vi "Wait For Motion Done.vi"(8 "error in (no error)":errorcluster, 9 "Mono2 Motor Pos":refnum<vi>, 10 "Axis":i32=1, 11 "VISA resource name":refnum<visa-resource-name>) -> (0 "error out":errorcluster, 3 "VISA resource name out":refnum<visa-resource-name>)   [LabVIEW 2019]
panel:
  in  "Mono2 Motor Pos":dbl caption="Motor Pos"
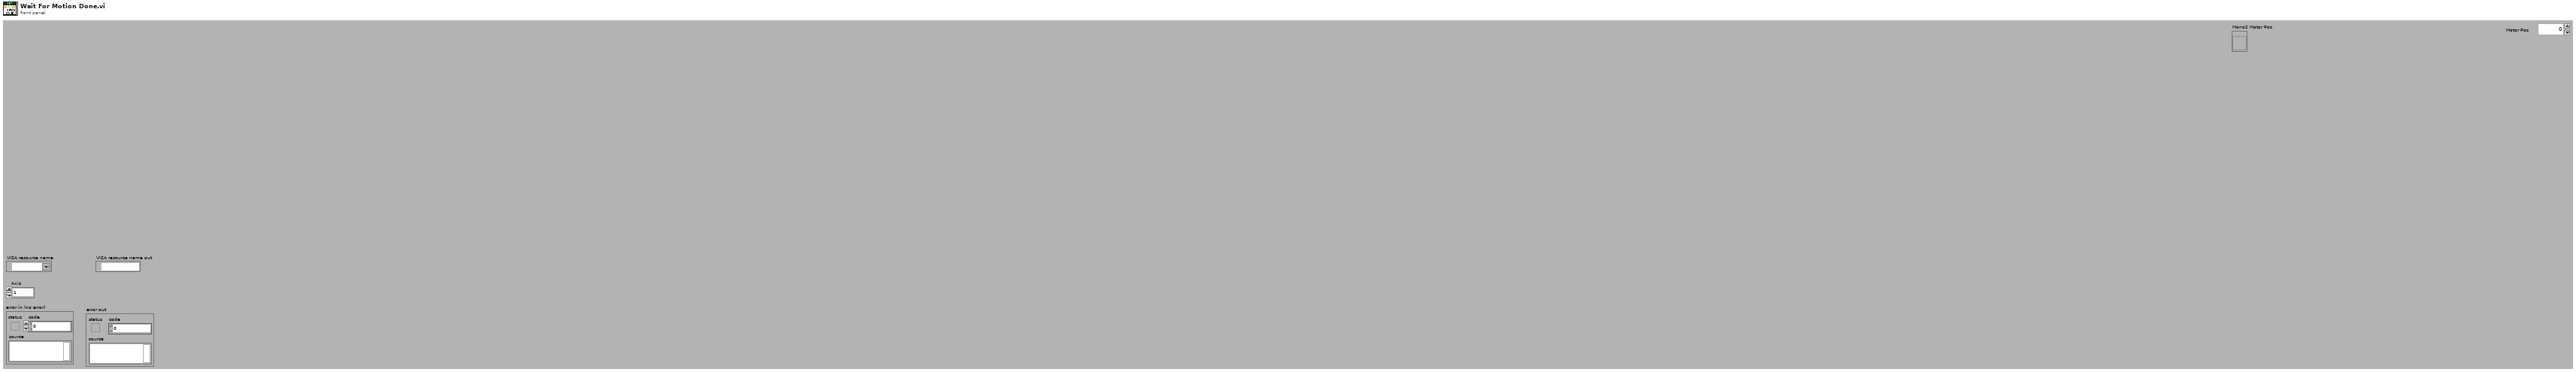
[diagram p1: front panel]
types:
  T1 = enum8{"Enabled", "Disabled", "Disabled and Grayed Out"}
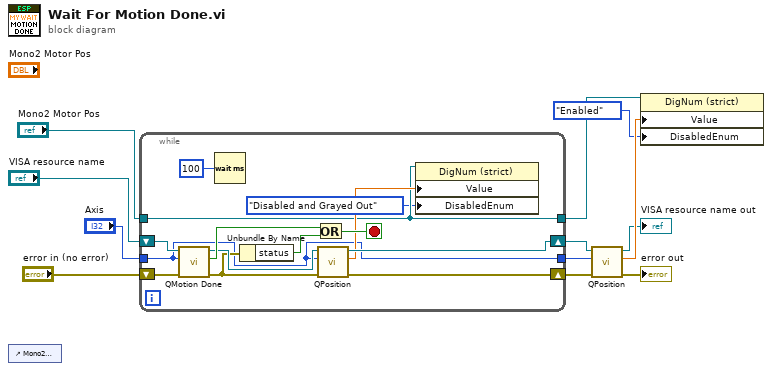
[diagram p0: block diagram]
diagram:
  n1 = control-ref of="Mono2 Motor Pos"() -> ()  [unwired: 1 out]
  n2 = while {
    shift-right: [w19] -> w4
    shift-left: "VISA resource name" -> [w26]
    shift-right: [w17] -> w7
    shift-left: "error in (no error)" -> [w25]
    tunnel: "Axis" -> [w15]
    tunnel: [w15] -> w8
    tunnel: [w14] -> w3
    tunnel: "Mono2 Motor Pos" -> [w14]
    stop <- w22 stop-if-true
    n3 = call "QMotion Done.vi"("error in (no error)"=w25, "Axis"=w15, "VISA resource name in"=w26) -> ("error out"=w18:errorcluster, "Motion Done?"=w23:bool, "VISA resource name out"=w20:refnum<visa-resource-name>)  [unwired: 6 in]
    n4 = Wait (ms)(milliseconds to wait=u32 100) -> ()  [unwired: 1 out]
    n5 = Unbundle By Name(w18) -> ("status"=w24:bool)
    n6 = Or(x=w23, y=w24) -> (x .or. y?=w22:bool)
    n7 = call "QPosition.vi"("error in (no error)"=w18, "Axis"=w15, "VISA resource name in"=w20) -> ("error out"=w17:errorcluster, "Position"=w16:dbl, "VISA resource name out"=w19:refnum<visa-resource-name>)  [unwired: 6 in]
    n8 = property class="DigNum (strict)"(reference=w14, "Value"=w16, "DisabledEnum"=T1."Disabled and Grayed Out" ("Disabled")) -> ()  [unwired: 1 in, 2 out]
  }
  n9 = call "QPosition.vi"("error in (no error)"=w7, "Axis"=w8, "VISA resource name in"=w4) -> ("error out"=→"error out":errorcluster, "Position"=w9:dbl, "VISA resource name out"=→"VISA resource name out":refnum<visa-resource-name>)  [unwired: 6 in]
  n10 = property class="DigNum (strict)"(reference=w3, "Value"=w9, "DisabledEnum"=T1."Enabled" ("Disabled")) -> ()  [unwired: 1 in, 2 out]
